vi "Compensated Chirp Demo.vi"() -> ()   [LabVIEW 2015]
uses:
  Controls/Level XCtl/Level Modes.ctl
  Controls/Level XCtl/Level Data.ctl
  Controls/Level XCtl/Level XCtl.xctl
  Controls/Level XCtl/Level Units.ctl
  Waveform VIs/FM Sweep VIs/FM Sweep Params.ctl
panel:
  out "dB SPL":dbl
  out "Magnitude Spectrum":T1(graph)
  out "Max Level":dbl
  in  "FMSweep In":T2={"Rate (oct/s)"=42900000.0, "Fmin (Hz)"=100.0, "Fmax (Hz)"=60000.0, "Ramp (ms)"=0.1, "Linear"=TRUE}
  out "Waveform Graph":cluster{i32, "dx":dbl, "Array":dbl[]}[](graph)
  in  "Fs (Hz)":dbl=200000.0
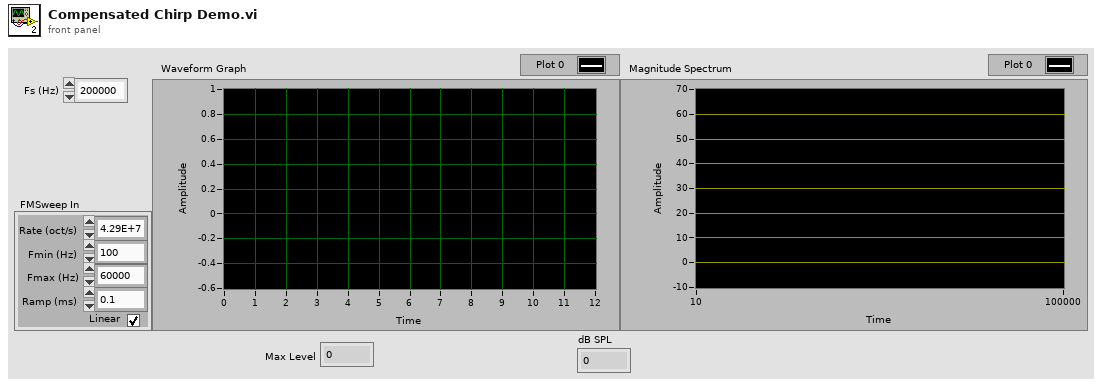
[diagram p1: front panel]
types:
  T1 = cluster{"Magnitude (dB)":dbl[], "Magnitude (dB)":dbl[]}
  T2 = typedef "FM Sweep Params.ctl" = cluster{"Rate (oct/s)":dbl, "Fmin (Hz)":dbl, "Fmax (Hz)":dbl, "Ramp (ms)":dbl, "Linear":bool}
  T3 = typedef "Level Modes.ctl" = enum16{"dB atten", "dB SPL", "dB re 1 Vrms", "dB V/Hz½"}
  T4 = typedef "Level XCtl.xctl/Level Data.ctl" = cluster{"Level":dbl, "Units":T5, "Max":dbl, "Multiplier":dbl, "Cal File":path, "Cal":cluster{"Freq (Hz)":dbl[], "Mag (dB SPL)":dbl[], "Phase (deg)":dbl[]}}
  T5 = typedef "Level Units.ctl" = enum16{"dB atten", "dB SPL", "dB re 1 Vrms", "dB V/Hz½", "mW", "dB SL"}
  T6 = cluster{"Freq (Hz)":dbl[], "Magnitude (dB)":dbl[]}
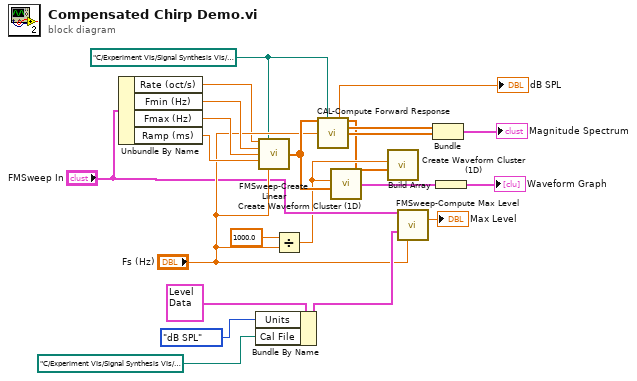
[diagram p0: block diagram]
diagram:
  w1 = path "C:/Experiment VIs/Signal Synthesis VIs/Test VIs/LeftPrimary.calib" ("Cal File")
  n1 = Unbundle By Name("FMSweep In") -> ("Rate (oct/s)"=w4:dbl, "Fmin (Hz)"=w9:dbl, "Fmax (Hz)"=w8:dbl, "Ramp (ms)"=w7:dbl)
  n2 = Bundle By Name(cluster=T4 {"Level"=0.0, "Units"=enum."dB atten", "Max"=0.0, "Multiplier"=0.0, "Cal File"=path "", "Cal"={"Freq (Hz)"=[], "Mag (dB SPL)"=[], "Phase (deg)"=[]}} ("Level"), "Units"=Level_Modes."dB SPL" ("Mode"), "Cal File"=path "C:/Experiment VIs/Signal Synthesis VIs/Test VIs/LeftPrimary.calib") -> (w19:T4)
  n3 = call "FMSweep-Create Linear.vi"("Sweep Rate (Hz/s)"=w4, "cal file"=w1, "Fmin (Hz)"=w9, "Fmax (Hz)"=w8, "Ramp (ms)"=w7, "Fs (Hz)"="Fs (Hz)") -> ("Array"=w10:dbl[])  [unwired: 7 in, 2 out]
  n4 = Divide(x=1000.0, y="Fs (Hz)") -> (x/y=w3:dbl)
  n5 = call "CAL-Compute Forward Response.vi"("Y"=w10, "Calibration file"=w1, "Fs (Hz)"="Fs (Hz)") -> ("dB SPL"=→"dB SPL":dbl, "Yfilt"=w2:dbl[], "Freq (Hz)"=w13:dbl[], "Magnitude (dB)"=w11:dbl[])  [unwired: 8 in, 1 out]
  n6 = call "Create Waveform Cluster (1D).vi"("Array"=w10, "dx"=w3) -> ("waveform cluster"=w15:cluster{i32, "dx":dbl, "Array":dbl[]})  [unwired: 2 in]
  n7 = call "Create Waveform Cluster (1D).vi"("Array"=w2, "dx"=w3) -> ()  [unwired: 2 in, 1 out]
  n8 = call "FMSweep-Compute Max Level.vi"("FMSweep"="FMSweep In", "Level"=w19, "Fs (Hz)"="Fs (Hz)") -> ("Max Level"=→"Max Level":dbl)  [unwired: 10 in, 2 out]
  n9 = Bundle("Freq (Hz)"=w13, "Magnitude (dB)"=w11) -> (→"Magnitude Spectrum":T6)  [unwired: 1 in]
  n10 = Build Array(w15) -> (→"Waveform Graph":cluster{i32, "dx":dbl, "Array":dbl[]}[])
